vi "Untitleds 2 (SubVI).vi"(8 "Fuel Type":bool, 9 "T2":dbl, 11 "stoic":dbl) -> (0 "gamma g":dbl, 3 "cpg":dbl)   [LabVIEW 2019]
panel:
  out "h":dbl
  out "g":dbl
  out "f":dbl
  out "e":dbl
  out "d":dbl
  out "c":dbl
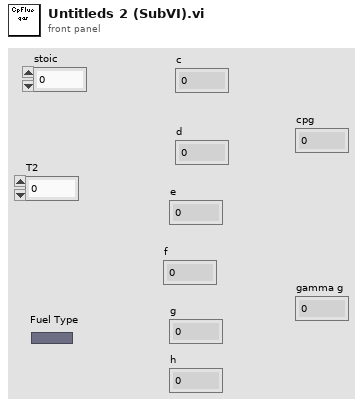
[diagram p1: front panel]
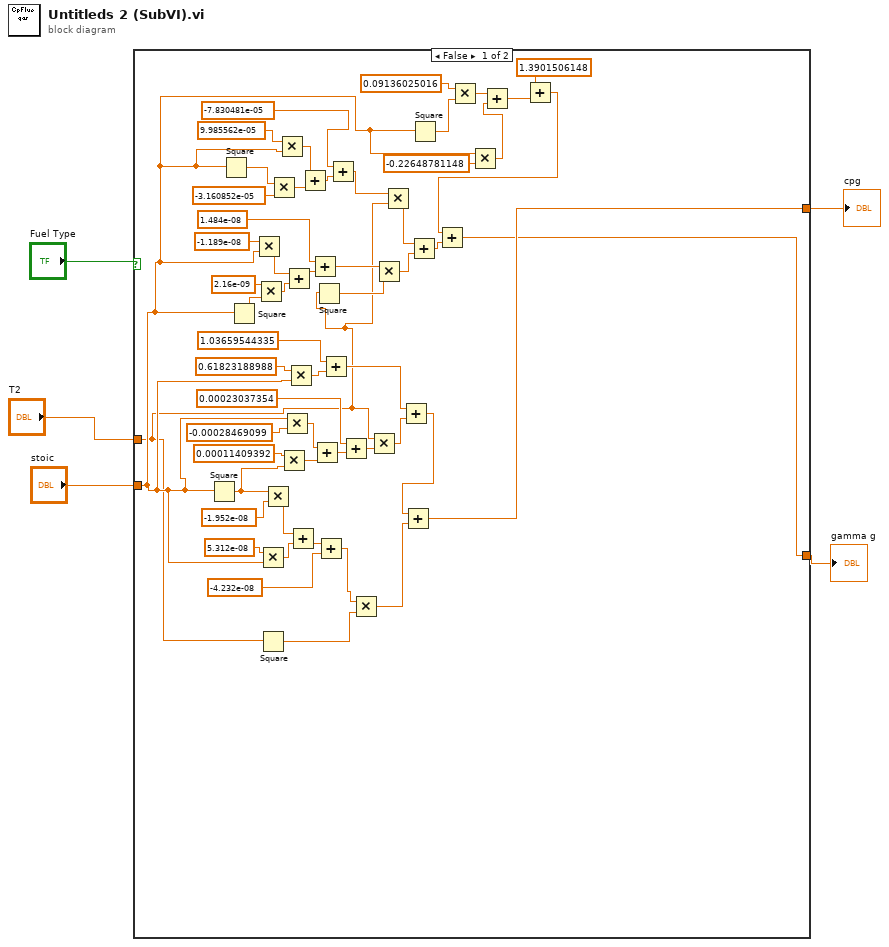
[diagram p0: block diagram]
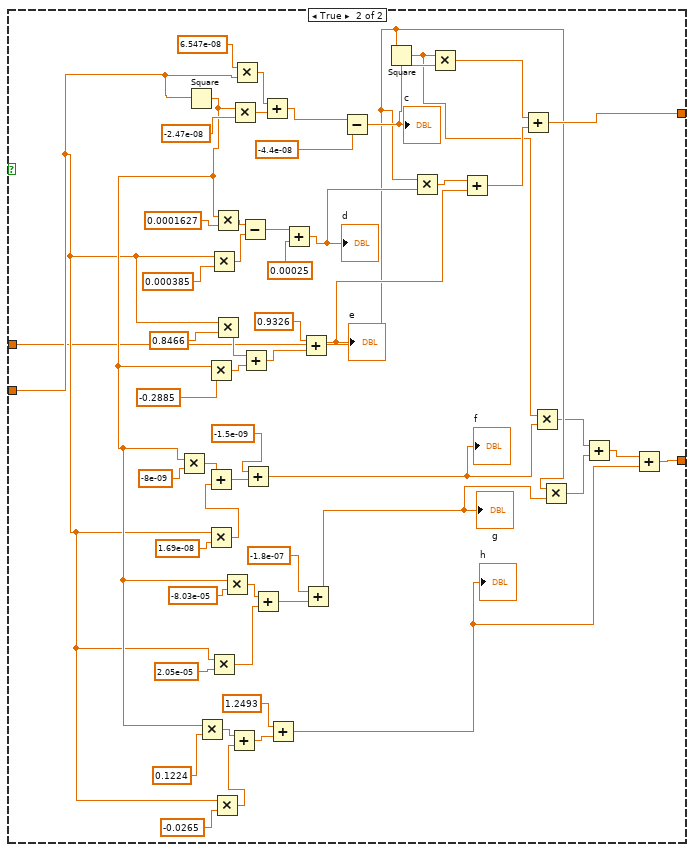
[diagram p2: hidden frame]
diagram:
  n1 = case shown="False" "Fuel Type" {
    tunnel: [w37 w90] -> w5
    tunnel: "stoic" -> [w18 w73]
    tunnel: "T2" -> [w11 w66]
    tunnel: [w6 w61] -> w2
    frame False {
      n2 = Square(x=w18) -> (x^2=w53:dbl)
      n3 = Square(x=w18) -> (x^2=w28:dbl)
      n4 = Square(x=w18) -> (x^2=w35:dbl)
      n5 = Multiply(x=-1.189e-08, y=w18) -> (x*y=w33:dbl)
      n6 = Multiply(x=2.16e-09, y=w35) -> (x*y=w34:dbl)
      n7 = Multiply(x=5.312e-08, y=w18) -> (x*y=w58:dbl)
      n8 = Square(x=w11) -> (x^2=w43:dbl)
      n9 = Multiply(x=w53, y=-1.952e-08) -> (x*y=w57:dbl)
      n10 = Multiply(x=w28, y=-3.160852e-05) -> (x*y=w27:dbl)
      n11 = Multiply(x=9.985562e-05, y=w18) -> (x*y=w26:dbl)
      n12 = Multiply(x=0.00011409392, y=w53) -> (x*y=w52:dbl)
      n13 = Multiply(x=w18, y=-0.00028469099) -> (x*y=w51:dbl)
      n14 = Add(x=w33, y=w34) -> (x+y=w31:dbl)
      n15 = Multiply(x=0.61823188988, y=w18) -> (x*y=w46:dbl)
      n16 = Add(x=w57, y=w58) -> (x+y=w56:dbl)
      n17 = Add(x=w26, y=w27) -> (x+y=w24:dbl)
      n18 = Add(x=1.484e-08, y=w31) -> (x+y=w14:dbl)
      n19 = Add(x=w51, y=w52) -> (x+y=w49:dbl)
      n20 = Square(x=w11) -> (x^2=w13:dbl)
      n21 = Add(x=w56, y=-4.232e-08) -> (x+y=w44:dbl)
      n22 = Add(x=1.03659544335, y=w46) -> (x+y=w40:dbl)
      n23 = Add(x=-7.830481e-05, y=w24) -> (x+y=w12:dbl)
      n24 = Add(x=0.00023037354, y=w49) -> (x+y=w42:dbl)
      n25 = Multiply(x=w44, y=w43) -> (x*y=w39:dbl)
      n26 = Multiply(x=w11, y=w42) -> (x*y=w41:dbl)
      n27 = Multiply(x=w14, y=w13) -> (x*y=w10:dbl)
      n28 = Multiply(x=w12, y=w11) -> (x*y=w9:dbl)
      n29 = Add(x=w40, y=w41) -> (x+y=w38:dbl)
      n30 = Add(x=w38, y=w39) -> (x+y=w37:dbl)
      n31 = Add(x=w9, y=w10) -> (x+y=w8:dbl)
      n32 = Square(x=w18) -> (x^2=w21:dbl)
      n33 = Multiply(x=0.09136025016, y=w21) -> (x*y=w20:dbl)
      n34 = Multiply(x=w18, y=-0.22648781148) -> (x*y=w17:dbl)
      n35 = Add(x=w20, y=w17) -> (x+y=w16:dbl)
      n36 = Add(x=1.3901506148, y=w16) -> (x+y=w7:dbl)
      n37 = Add(x=w7, y=w8) -> (x+y=w6:dbl)
    }
    frame True {
      n38 = Square(x=w73) -> (x^2=w77:dbl)
      n39 = Multiply(x=w77, y=-8e-09) -> (x*y=w88:dbl)
      n40 = Multiply(x=w77, y=0.1224) -> (x*y=w75:dbl)
      n41 = Multiply(x=w77, y=-0.2885) -> (x*y=w101:dbl)
      n42 = Multiply(x=w73, y=1.69e-08) -> (x*y=w86:dbl)
      n43 = Add(x=w88, y=w86) -> (x+y=w85:dbl)
      n44 = Multiply(x=w73, y=0.000385) -> (x*y=w106:dbl)
      n45 = Multiply(x=w73, y=2.05e-05) -> (x*y=w80:dbl)
      n46 = Multiply(x=w73, y=-0.0265) -> (x*y=w74:dbl)
      n47 = Multiply(x=w77, y=0.0001627) -> (x*y=w107:dbl)
      n48 = Multiply(x=w73, y=0.8466) -> (x*y=w99:dbl)
      n49 = Multiply(x=w77, y=-8.03e-05) -> (x*y=w82:dbl)
      n50 = Add(x=w75, y=w74) -> (x+y=w71:dbl)
      n51 = Multiply(x=w77, y=-2.47e-08) -> (x*y=w113:dbl)
      n52 = Multiply(x=6.547e-08, y=w73) -> (x*y=w112:dbl)
      n53 = Subtract(x=w107, y=w106) -> (x-y=w104:dbl)
      n54 = Add(x=w99, y=w101) -> (x+y=w98:dbl)
      n55 = Add(x=-1.5e-09, y=w85) -> (x+y=w69:dbl)
      "f" <- w69
      n56 = Add(x=w82, y=w80) -> (x+y=w79:dbl)
      n57 = Add(x=w112, y=w113) -> (x+y=w110:dbl)
      n58 = Add(x=1.2493, y=w71) -> (x+y=w63:dbl)
      "h" <- w63
      n59 = Add(x=w104, y=0.00025) -> (x+y=w95:dbl)
      "d" <- w95
      n60 = Add(x=0.9326, y=w98) -> (x+y=w94:dbl)
      "e" <- w94
      n61 = Add(x=-1.8e-07, y=w79) -> (x+y=w67:dbl)
      "g" <- w67
      n62 = Subtract(x=w110, y=-4.4e-08) -> (x-y=w96:dbl)
      "c" <- w96
      n63 = Square(x=w66) -> (x^2=w68:dbl)
      n64 = Multiply(x=w66, y=w95) -> (x*y=w93:dbl)
      n65 = Multiply(x=w68, y=w96) -> (x*y=w91:dbl)
      n66 = Add(x=w93, y=w94) -> (x+y=w92:dbl)
      n67 = Add(x=w91, y=w92) -> (x+y=w90:dbl)
      n68 = Multiply(x=w68, y=w69) -> (x*y=w65:dbl)
      n69 = Multiply(x=w66, y=w67) -> (x*y=w64:dbl)
      n70 = Add(x=w65, y=w64) -> (x+y=w62:dbl)
      n71 = Add(x=w62, y=w63) -> (x+y=w61:dbl)
    }
  }
  "cpg" <- w5
  "gamma g" <- w2
